vi "LV Client Test.vi"() -> ()   [LabVIEW 2018]
panel:
  out "Requests Sent":i32
  in  "stop":bool
  in  "Send Request":bool
  out "Data Response":u8[](array[numeric])
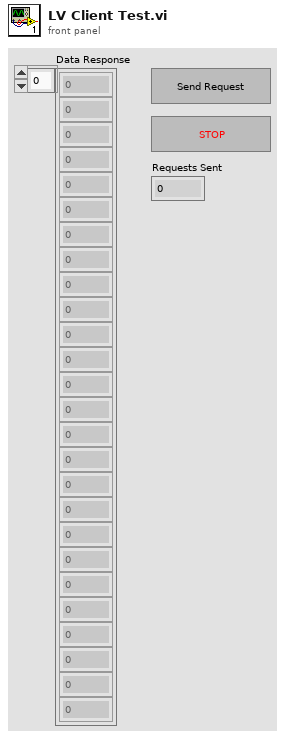
[diagram p1: front panel]
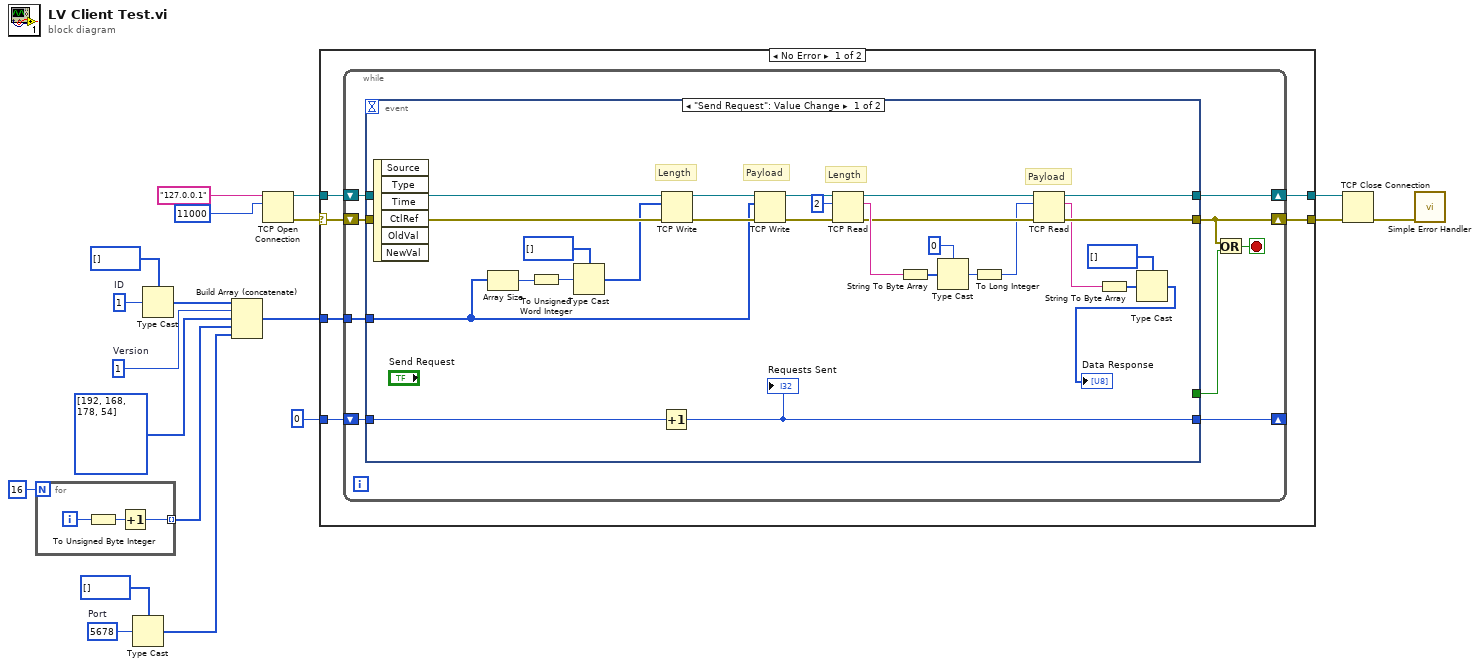
[diagram p0: block diagram]
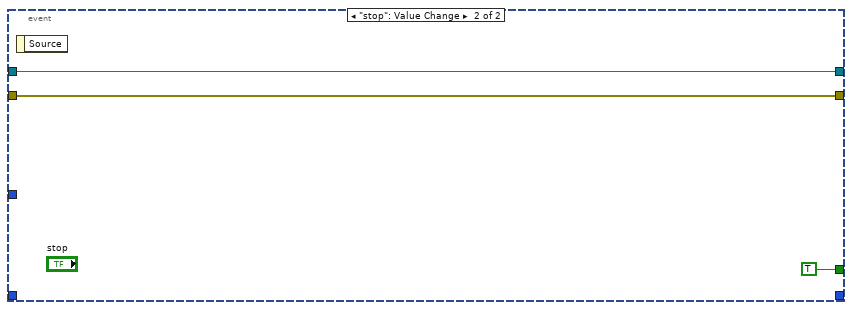
[diagram p2: hidden frame]
diagram:
  w8 = u16 5678  # Port
  w6 = u8 1  # Version
  w3 = u16 1  # ID
  n1 = for {
    N: 16 -> [_]
    tunnel: [w21] -> w10 mode=indexing
    i -> [w22]
    n2 = To Unsigned Byte Integer(number=w22) -> (unsigned 8bit integer=w20:u8)
    n3 = Increment(x=w20) -> (x+1=w21:u8)
  }
  n4 = Type Cast(type=u8[] [], x=w8) -> (*(type *) &x=w11:u8[])
  n5 = Type Cast(type=u8[] [], x=w3) -> (*(type *) &x=w9:u8[])
  n6 = Build Array (concatenate)(w9, w6, u8[] [192, 168, 178, 54], w10, w11) -> (w1:u8[])
  n7 = TCP Open Connection(address="127.0.0.1", remote port or service name=u16 11000) -> (connection ID=w19:refnum<k5>, error out=w18:errorcluster)  [unwired: 3 in]
  n8 = case shown="No Error" w18 {
    selector: w18 -> [w27 w68]
    tunnel: w19 -> [w28 w69]
    tunnel: [w26 w69] -> w15
    tunnel: [w25 w68] -> w14
    tunnel: 0 -> [w24 _]
    tunnel: w1 -> [w23 _]
    frame No Error {
      n9 = while {
        shift-right: [w35] -> w26
        shift-left: w28 -> [w37]
        shift-right: [w31] -> w25
        shift-left: w27 -> [w36]
        shift-right: [w32] -> _
        shift-left: w24 -> [w33]
        tunnel: w23 -> [w34]
        stop <- w29 stop-if-true
        n10 = event shown="[0] \"Send Request\": Value Change" {
          selector: _ -> [_ _]
          dyn-events: _ -> [_ _]
          timeout: _ -> [_ _]
          tunnel: w37 -> [w64 w67]
          tunnel: w36 -> [w63 w66]
          tunnel: [w49 w67] -> w35
          tunnel: [w48 w66] -> w31
          tunnel: [_ TRUE] -> w30
          tunnel: w34 -> [w40 _]
          tunnel: w33 -> [w39 _]
          tunnel: [w38 _] -> w32
          event "Send Request": Value Change {
            # "Payload"
            # "Length"
            # "Payload"
            # "Length"
            n11 = event-data() -> ()  [unwired: 1 in, 6 out]
            n12 = Array Size(array=w40) -> (size(s)=w60:i32)
            n13 = To Unsigned Word Integer(number=w60) -> (unsigned 16bit integer=w59:u16)
            n14 = Type Cast(type=u8[] [], x=w59) -> (*(type *) &x=w57:u8[])
            n15 = Increment(x=w39) -> (x+1=w38:i32)
            "Requests Sent" <- w38
            n16 = TCP Write(connection ID=w64, data in=w57, error in (no error)=w63) -> (connection ID out=w62:refnum<k5>, error out=w61:errorcluster)  [unwired: 1 in, 1 out]
            n17 = TCP Write(connection ID=w62, data in=w40, error in (no error)=w61) -> (connection ID out=w56:refnum<k5>, error out=w55:errorcluster)  [unwired: 1 in, 1 out]
            n18 = TCP Read(connection ID=w56, bytes to read=2, error in (no error)=w55) -> (connection ID out=w51:refnum<k5>, data out=w53:string, error out=w50:errorcluster)  [unwired: 2 in]
            n19 = String To Byte Array(string=w53) -> (unsigned byte array=w52:u8[])
            n20 = Type Cast(type=u16 0, x=w52) -> (*(type *) &x=w43:u16)
            n21 = To Long Integer(number=w43) -> (32bit integer=w42:i32)
            n22 = TCP Read(connection ID=w51, bytes to read=w42, error in (no error)=w50) -> (connection ID out=w49:refnum<k5>, data out=w45:string, error out=w48:errorcluster)  [unwired: 2 in]
            n23 = String To Byte Array(string=w45) -> (unsigned byte array=w46:u8[])
            n24 = Type Cast(type=u8[] [], x=w46) -> (*(type *) &x=→"Data Response":u8[])
          }
          event "stop": Value Change {
            n25 = event-data() -> ()  [unwired: 1 in, 1 out]
          }
        }
        n26 = Or(x=w31, y=w30) -> (x .or. y?=w29:bool)
      }
    }
    frame Error {
    }
  }
  n27 = TCP Close Connection(connection ID=w15, error in (no error)=w14) -> (error out=w13:errorcluster)  [unwired: 1 in, 1 out]
  n28 = call <vilib>:"Simple Error Handler.vi"("error in (no error)"=w13) -> ()  [unwired: 4 in, 5 out]
